vi "Update Property by Name.vi"(8 "error in (no error)":errorcluster, 9 "Value":variant, 10 "Name":string, 11 "ColumnPanel in":refnum<class "ColumnPanel.lvclass">) -> (0 "error out":errorcluster, 3 "ColumnPanel out":refnum<class "ColumnPanel.lvclass">)   [LabVIEW 2020, in "Conditum-Tools.lvlib" / "ColumnPanel.lvclass"]
uses:
  ColumnPanel.lvclass
  Property Update.ctl
  ColumnPanel.lvclass/ColumnPanel.ctl
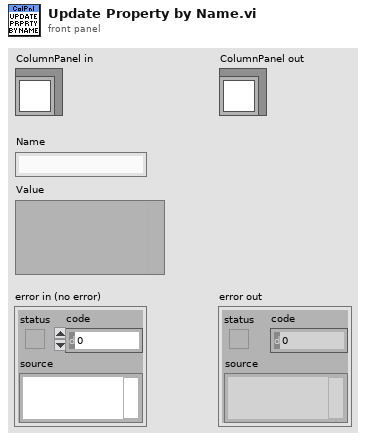
[diagram p1: front panel]
types:
  T1 = typedef "Conditum-Tools.lvlib/ColumnPanel.lvclass/Property Update.ctl" = cluster{"Name":string, "Value":variant}
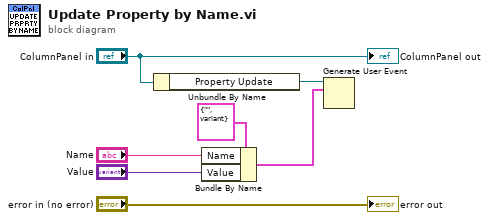
[diagram p0: block diagram]
diagram:
  n1 = Unbundle By Name("ColumnPanel in") -> ("Property Update"=w5:refnum<user-event>)
  n2 = Bundle By Name(cluster=T1 {"Name"="", "Value"=variant} ("Property Update"), "Name"="Name", "Value"="Value") -> (w4:T1)
  n3 = Generate User Event(user event=w5, event data cluster=w4) -> ()  [unwired: 2 in, 2 out]
  "error out" <- "error in (no error)"
  "ColumnPanel out" <- "ColumnPanel in"
